vi "setUp.vi"(8 "error in (no error)":errorcluster, 11 "reference in":refnum<class "MixedTest TestSuite.lvclass">) -> (0 "error out":errorcluster, 3 "reference out":refnum<class "MixedTest TestSuite.lvclass">)   [LabVIEW 2011, in "MixedTest TestSuite.lvclass"]
uses:
  MixedTest TestSuite.lvclass
  MixedTest TestSuite.lvclass/MixedTest TestSuite.ctl
  Classes/TestSuite/TestSuite.lvclass
panel:
  out "created new?":bool
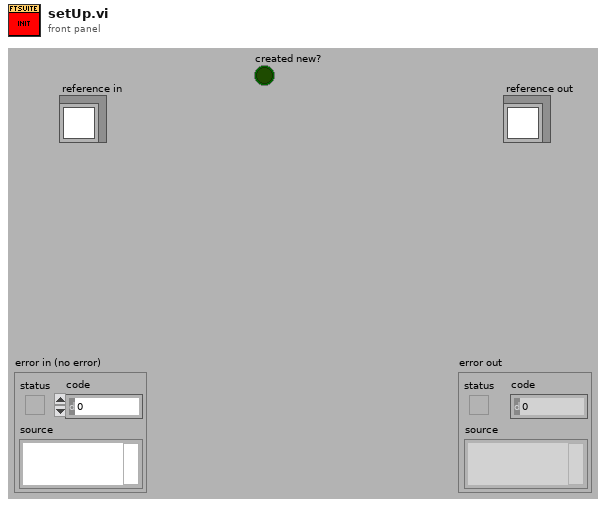
[diagram p1: front panel]
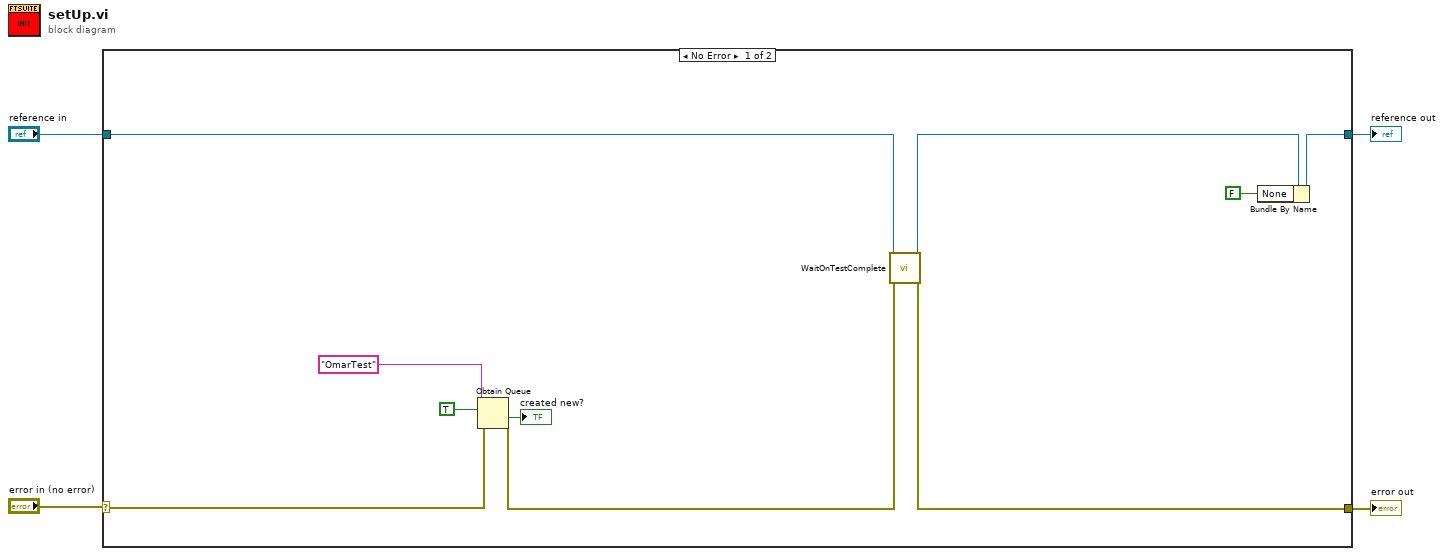
[diagram p0: block diagram]
diagram:
  n1 = case shown="No Error" "error in (no error)" {
    selector: "error in (no error)" -> [w12 w15]
    tunnel: [w14 w16] -> w4
    tunnel: "reference in" -> [w8 w16]
    tunnel: [w5 w15] -> w1
    frame No Error {
      n2 = Obtain Queue(name (unnamed)="OmarTest", element data type=TRUE, error in (no error)=w12) -> (created new?=→"created new?":bool, error out=w6:errorcluster)  [unwired: 2 in, 1 out]
      n3 = call "WaitOnTestComplete.vi"("error in (no error)"=w6, "TestSuite in"=w8) -> ("error out"=w5:errorcluster, "TestSuite out"=w7:refnum<class "MixedTest TestSuite.lvclass">)  [unwired: 8 in]
      n4 = Bundle By Name(cluster=w7, "None"=FALSE) -> (w14:refnum<class "MixedTest TestSuite.lvclass">)
    }
    frame Error {
    }
  }
  "reference out" <- w4
  "error out" <- w1
